vi "UserManager_GetAttributes.vi"(8 "ErrorIn":errorcluster, 10 "OnlyGetDvrReference(False)":bool, 11 "ReferenceIn":refnum<class "UserManager.lvclass">) -> (0 "ErrorOut":errorcluster, 1 "DataRef":refnum<data-value>, 2 "Data":T1, 3 "ReferenceOut":refnum<class "UserManager.lvclass">)   [LabVIEW 2021, in "UserMananger.lvlib" / "UserManager.lvclass"]
uses:
  UserManager.lvclass
  protected/ObjectAttributes.ctl
  Interface_TAF_AutorizationUpdated/IAuthorizationUpdated/IAuthorizationUpdated.lvclass
  UserManager.lvclass/UserManager.ctl
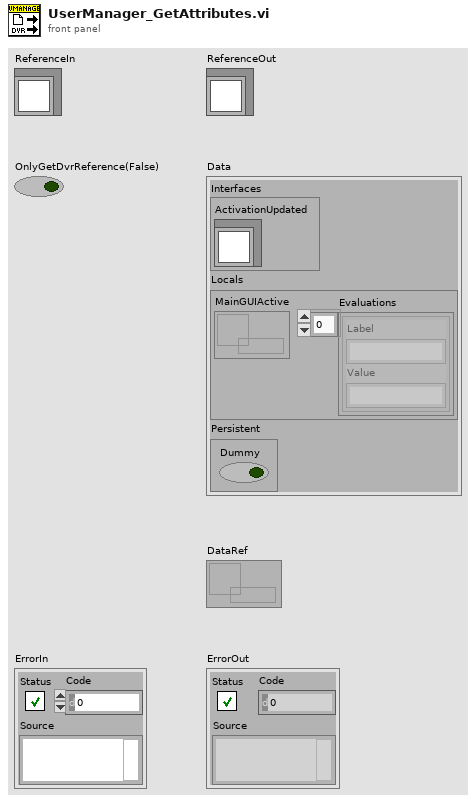
[diagram p1: front panel]
types:
  T1 = typedef "UserMananger.lvlib/UserManager.lvclass/ObjectAttributes.ctl" = cluster{"Interfaces":cluster{"ActivationUpdated":refnum<class "IAuthorizationUpdated.lvclass">}, "Locals":cluster{"MainGUIActive":refnum<queue>, "Evaluations":cluster{"Label":string, "Value":string}[]}, "Persistent":cluster{"Dummy":bool}}
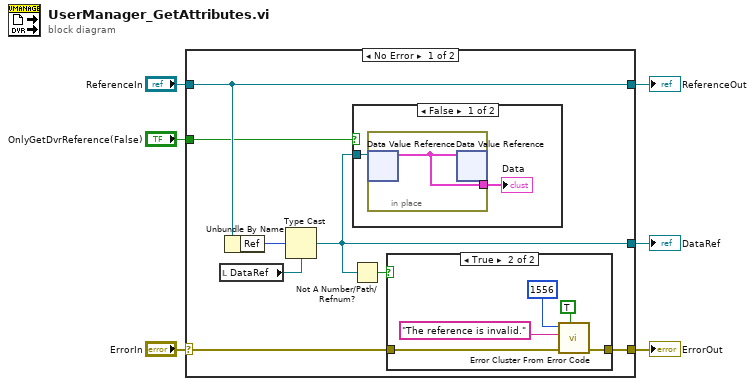
[diagram p0: block diagram]
diagram:
  n1 = case shown="No Error" "ErrorIn" {
    selector: "ErrorIn" -> [w14 w25]
    tunnel: [w13 w25] -> w5
    tunnel: [w12 w24] -> w3
    tunnel: "ReferenceIn" -> [w12 w24]
    tunnel: [w7 _] -> w2
    tunnel: "OnlyGetDvrReference(False)" -> [w9 _]
    frame No Error {
      n2 = local read "DataRef"() -> (w10:refnum<data-value>)
      n3 = Unbundle By Name(w12) -> ("Ref"=w11:u32)
      n4 = Type Cast(type=w10, x=w11) -> (*(type *) &x=w7:refnum<data-value>)
      n5 = Not A Number/Path/Refnum?(number/path/refnum=w7) -> (NaN/Path/Refnum?=w8:bool)
      n6 = case shown="False" w9 {
        tunnel: w7 -> [w22 _]
        frame False {
          n7 = in-place {
            in-place-border: [w23] -> w21
            n8 = in-place-dvr #1(w22) -> (w23:T1)  [unwired: 1 out]
            n9 = in-place-dvr #1(w23) -> ()  [unwired: 2 out]
          }
          "Data" <- w21
        }
        frame True {
        }
      }
      n10 = case shown="True" w8 {
        tunnel: w14 -> [w15 w20]
        tunnel: [w15 w19] -> w13
        frame False {
        }
        frame True {
          n11 = call <vilib>:"Error Cluster From Error Code.vi"("show call chain? (False)"=TRUE, "error in (no error)"=w20, "error message (\"\")"="The reference is invalid." ("source"), "error code (0)"=1556 ("code")) -> ("error out"=w19:errorcluster)  [unwired: 5 in]
        }
      }
    }
    frame Error {
    }
  }
  "ErrorOut" <- w5
  "ReferenceOut" <- w3
  "DataRef" <- w2
